vi "Scale Data.vi"(0 "reference in":refnum<class "AD.lvclass">, 1 "Raw Data":dbl, 5 "error in (no error)":errorcluster) -> (14 "reference out":refnum<class "AD.lvclass">, 15 "Scaled Data":dbl, 19 "error out":errorcluster)   [LabVIEW 2013, in "AD.lvclass"]
uses:
  AD.lvclass
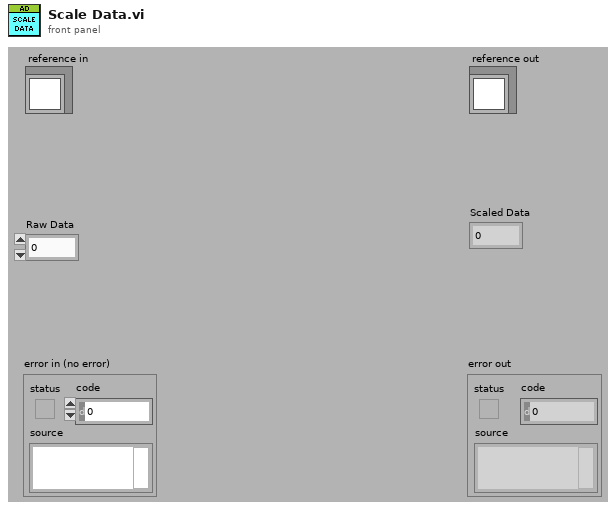
[diagram p1: front panel]
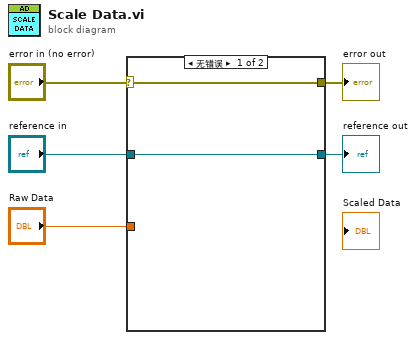
[diagram p0: block diagram]
diagram:
  n1 = case shown="无错误" "error in (no error)" {
    selector: "error in (no error)" -> [w6 w9]
    tunnel: [w6 w9] -> w4
    tunnel: [w7 w8] -> w2
    tunnel: "reference in" -> [w7 w8]
    tunnel: "Raw Data" -> [_ _]
    frame No Error {
    }
    frame Error {
    }
  }
  "error out" <- w4
  "reference out" <- w2
